vi "SVN_Info_SingleLogEntry_ParseCMDOutput.vi"(8 "Error In":errorcluster, 11 "SVN_Log_XML (In)":string="<?xml version=\"1.0\" encoding=\"UTF-8\"?>\r\n<log>\r\n<logentry\r\n   revision=\"23\">\r\n<author>Admin</author>\r\n<date>2018-04-07T20:16:29.107705Z</date>\r\n<msg></msg>\r\n</logentry>\r\n<logentry\r\n   revision=\"22\">\r\n<author>Admin</author>\r\n<date>2018-04-07T20:12:54.923454Z</date>\r\n<msg></msg>\r\n</logentry>\r\n<logentry\r\n   revision=\"21\">\r\n<author>Admin</author>\r\n<date>2018-04-07T20:12:03.070489Z</date>\r\n<msg></msg>\r\n</logentry>\r\n<logentry\r\n   revision=\"20\">\r\n<author>Marvin</author>\r\n<date>2017-12-05T21:00:12.256074Z</date>\r\n<msg></msg>\r\n</logentry>\r\n<logentry\r\n   revision=\"17\">\r\n<author>Marvin</author>\r\n<date>2017-12-05T20:36:10.326601Z</date>\r\n<msg>10k LoadSpeedTest\r\n</msg>\r\n</logentry>\r\n<logentry\r\n   revision=\"16\">\r\n<author>Marvin</author>\r\n<date>2017-07-06T14:47:03.129259Z</date>\r\n<msg></msg>\r\n</logentry>\r\n<logentry\r\n   revision=\"11\">\r\n<author>Marvin</author>\r\n<date>2017-07-04T16:12:46.837966Z</date>\r\n<msg></msg>\r\n</logentry>\r\n<logentry\r\n   revision=\"7\">\r\n<author>Marvin</author>\r\n<date>2017-07-04T16:05:39.382517Z</date>\r\n<msg></msg>\r\n</logentry>\r\n<logentry\r\n   revision=\"6\">\r\n<author>Marvin</author>\r\n<date>2017-07-04T16:05:05.356571Z</date>\r\n<msg></msg>\r\n</logentry>\r\n<logentry\r\n   revision=\"3\">\r\n<author>Marvin</author>\r\n<date>2017-07-04T15:57:28.132419Z</date>\r\n<msg></msg>\r\n</logentry>\r\n<logentry\r\n   revision=\"1\">\r\n<author>Marvin</author>\r\n<date>2017-07-04T15:51:57.071483Z</date>\r\n<msg>Imported folder structure</msg>\r\n</logentry>\r\n</log>\r\n") -> (0 "Error Out":errorcluster, 3 "SVN_Info_Cluster":T1)   [LabVIEW 2014]
uses:
  <resource>/objmgr/DOMUserDefRef.rc
  <vilib>/xml/NI_XML.lvlib
  <vilib>/xml/Load XML String.vi
  controls/SVN_LogEntry_Cluster.ctl
  controls/SVN_Info_Cluster.ctl
  <vilib>/xml/Close Reference(Node).vi
panel:
  out "commit node values this.Ver":string[](array[string])
  out "commit values this.Ver":string[](array[string])
  out "Attributes":string
  in  "XML String":string="<node_1>\n <node_2 name = \"second_node\"> text </node_2>\n <node_3 type = \"a\"> \n<node_4> text </node_4>\n </node_3>\n</node_1>"
  out "entry values HEAD":string[](array[string])
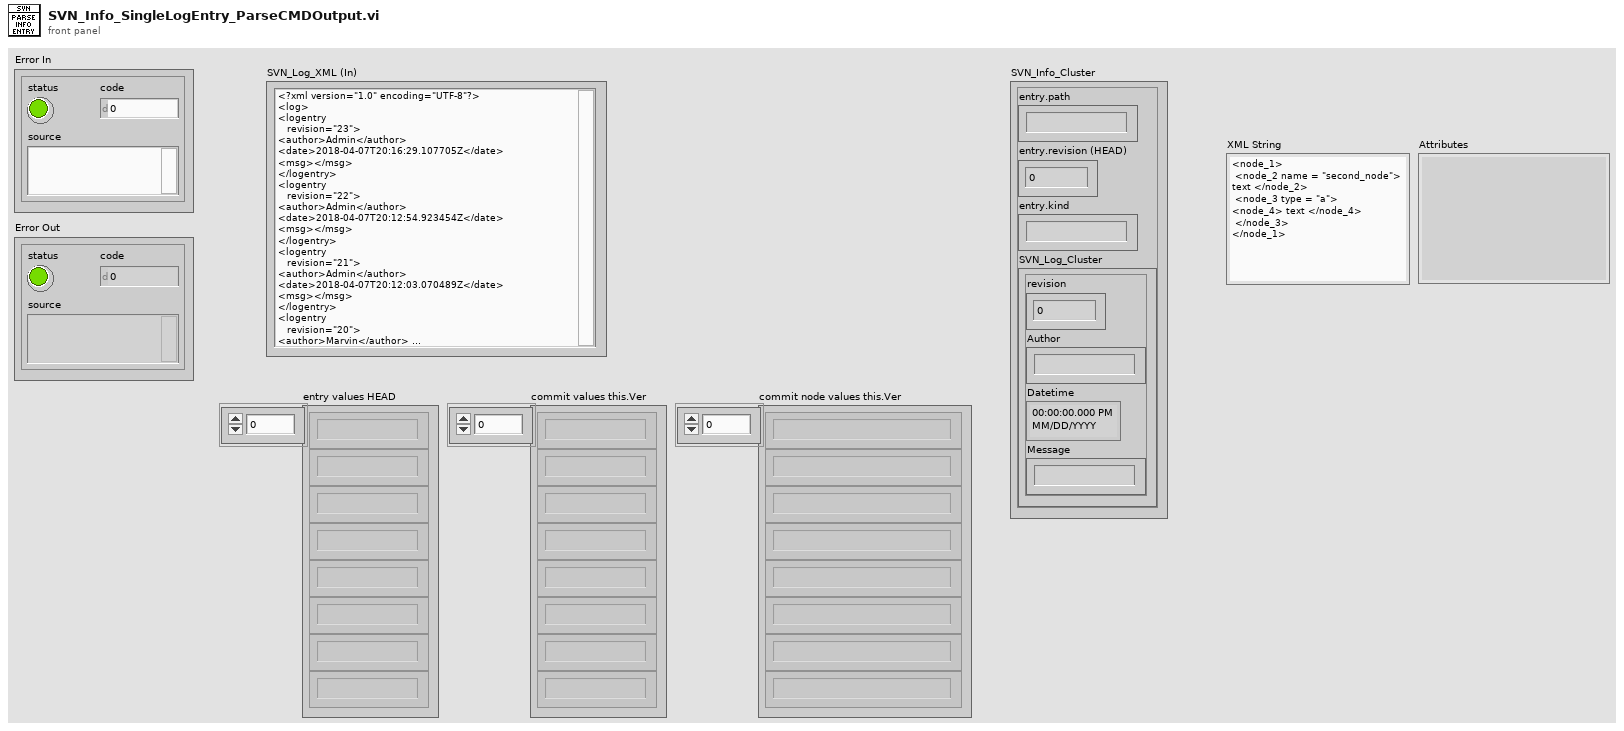
[diagram p1: front panel]
types:
  T1 = typedef "SVN_Info_Cluster.ctl" = cluster{"entry.path":string, "entry.revision (HEAD)":i32, "entry.kind":string, "SVN_Log_Cluster":T2}
  T2 = typedef "SVN_LogEntry_Cluster.ctl" = cluster{"revision":i32, "Author":string, "Datetime":timestamp, "Message":string}
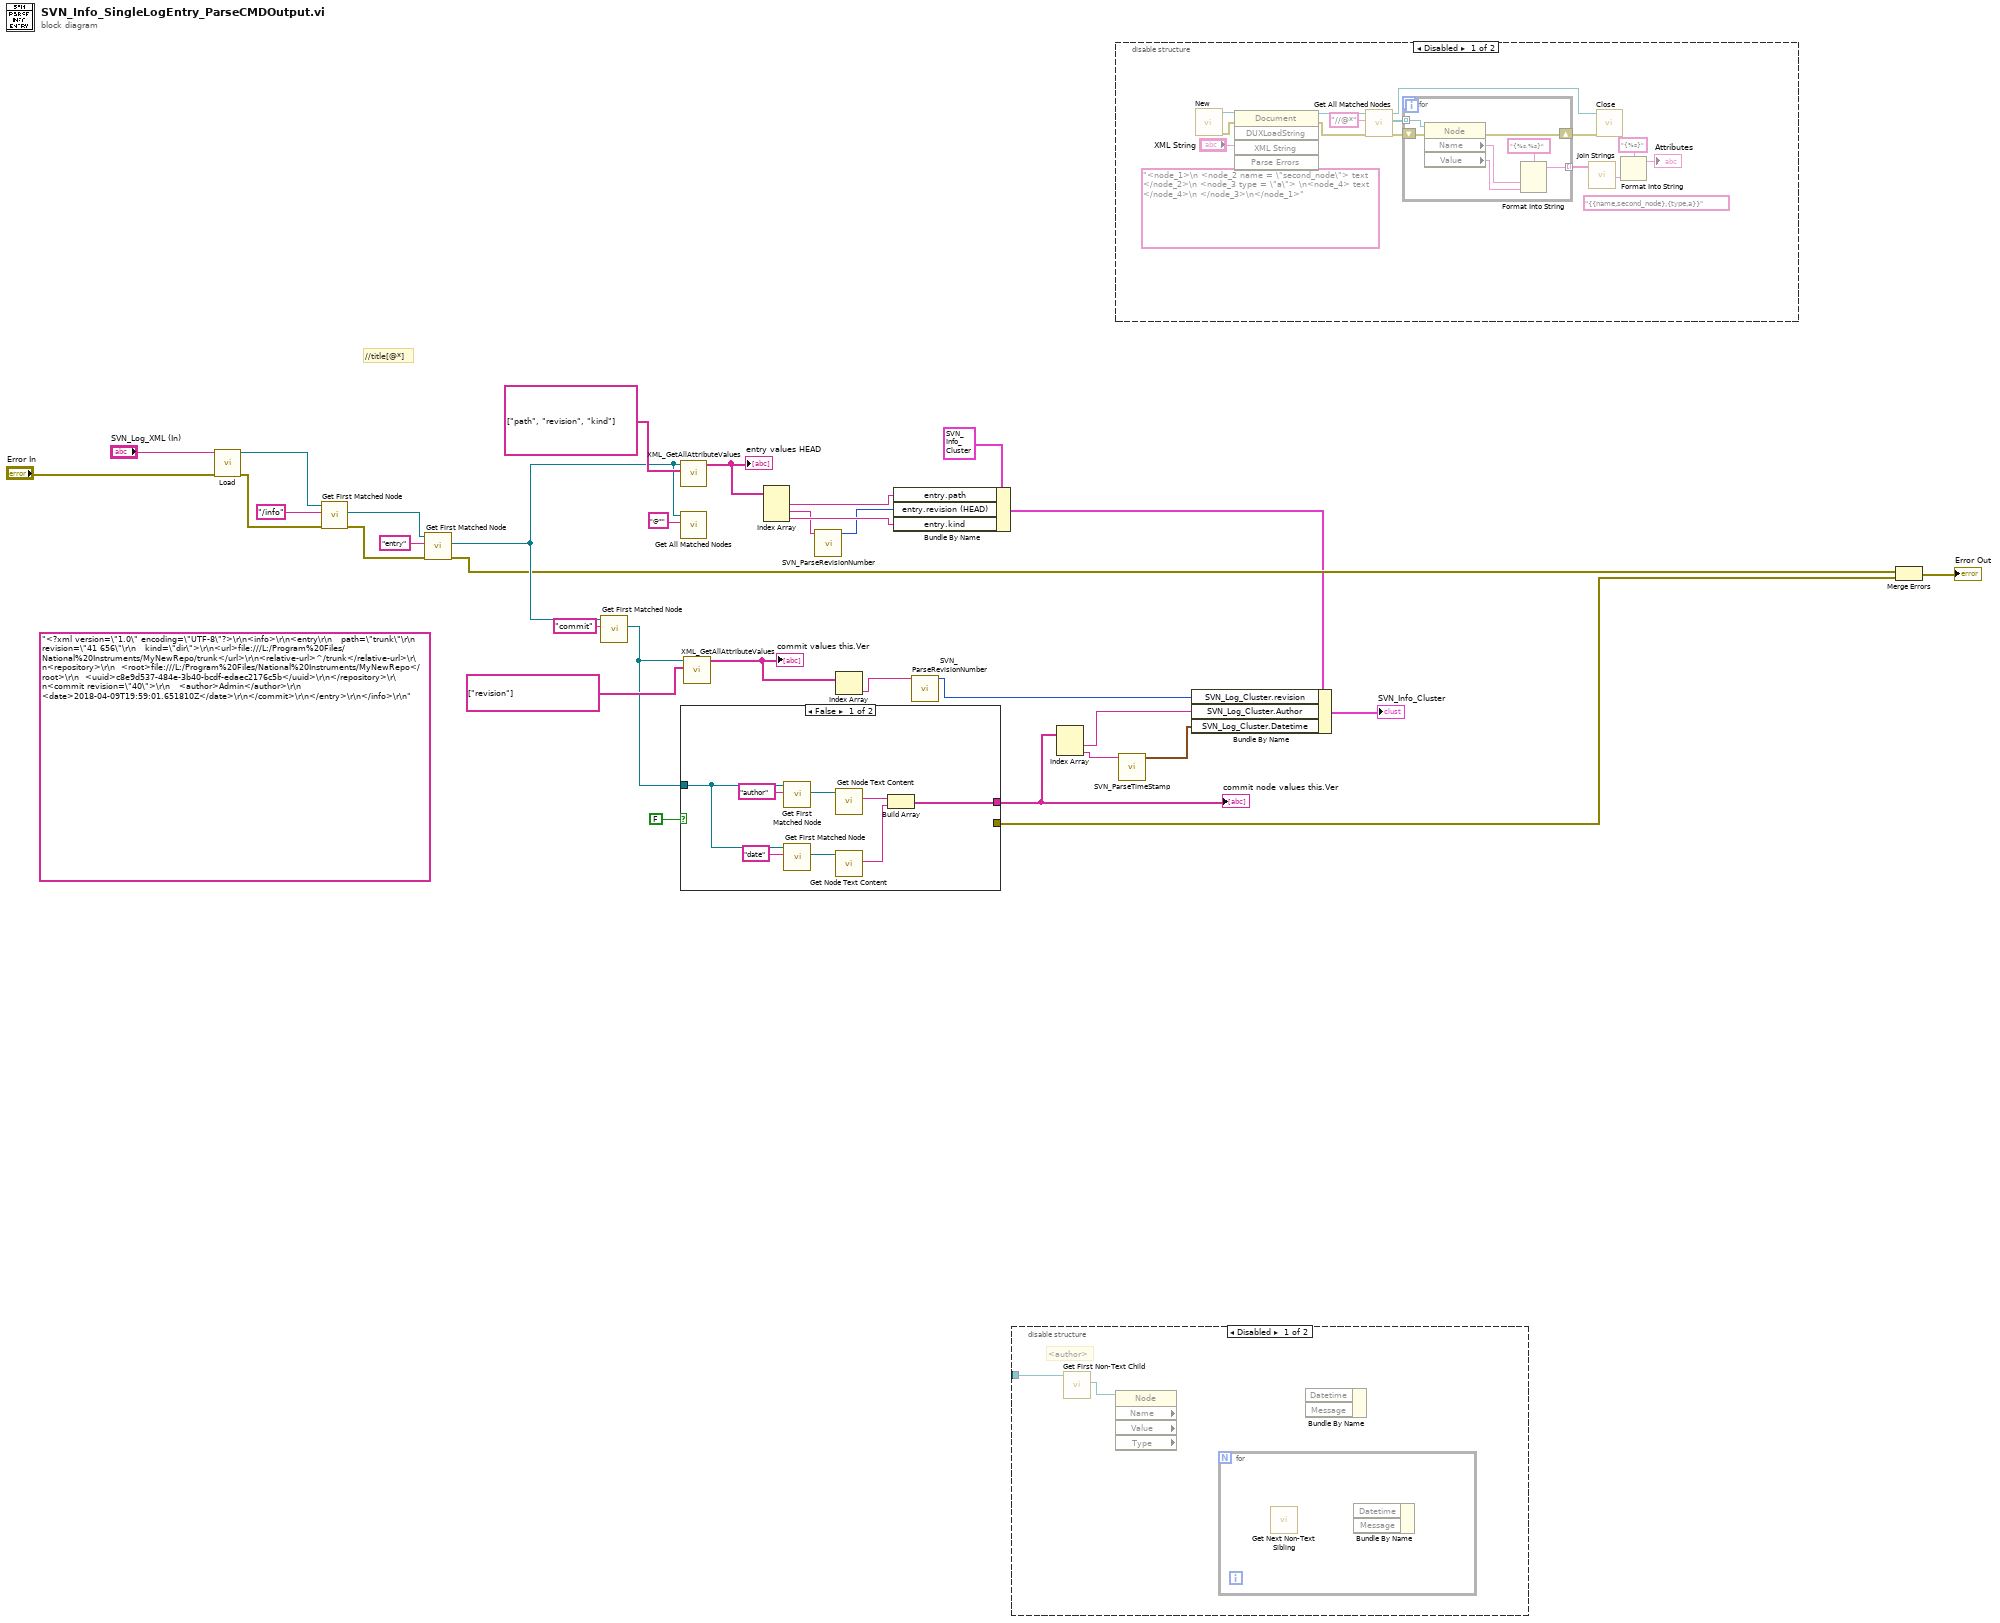
[diagram p0: block diagram]
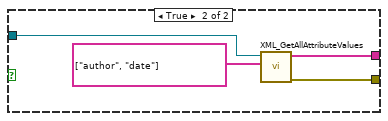
[diagram p2: hidden frame]
diagram:
  (unwired) "<?xml version=\"1.0\" encoding=\"UTF-8\"?>\r\n<info>\r\n<entry\r\n   path=\"trunk\"\r\n   revision=\"41 656\"\r\n   kind=\"dir\">\r\n<url>file:///L:/Program%20Files/National%20Instruments/MyNewRepo/trunk</url>\r\n<relative-url>^/trunk</relative-url>\r\n<repository>\r\n  <root>file:///L:/Program%20Files/National%20Instruments/MyNewRepo</root>\r\n  <uuid>c8e9d537-484e-3b40-bcdf-edaec2176c5b</uuid>\r\n</repository>\r\n<commit revision=\"40\">\r\n   <author>Admin</author>\r\n   <date>2018-04-09T19:59:01.651810Z</date>\r\n</commit>\r\n</entry>\r\n</info>\r\n"
  # "//title[@*]"
  n1 = call-poly <vilib>:"Load.vi"("XML string"="SVN_Log_XML (In)", "error in (no error)"="Error In") -> ("DOM document out"=w27:refnum<k20>, "error out"=w30:errorcluster)  [unwired: 11 in, 1 out]
  n2 = call <vilib>:"Get First Matched Node.vi"("error in (no error)"=w30, "XPath expression"="/info", "node in"=w27) -> ("error out"=w17:errorcluster, "node result"=w23:refnum<k20>)  [unwired: 6 in, 1 out]
  n3 = call <vilib>:"Get First Matched Node.vi"("error in (no error)"=w17, "XPath expression"="entry", "node in"=w23) -> ("error out"=w18:errorcluster, "node result"=w19:refnum<k20>)  [unwired: 6 in, 1 out]
  n4 = call <vilib>:"Get First Matched Node.vi"("XPath expression"="commit", "node in"=w19) -> ("node result"=w21:refnum<k20>)  [unwired: 7 in, 2 out]
  n5 = call "XML_GetAllAttributeValues.vi"("Attribute Names to find[]"=string[] ["path", "revision", "kind"], "Node Refnum (In)"=w19) -> ("Attribute Values[]"=w11:string[])  [unwired: 8 in, 1 out]
  "entry values HEAD" <- w11
  n6 = call <vilib>:"Get All Matched Nodes.vi"("XPath expression"="@*", "node in"=w19) -> ()  [unwired: 7 in, 3 out]
  n7 = case shown="False" FALSE {
    tunnel: w21 -> [w39 w45]
    tunnel: [w34 w44] -> w15
    tunnel: [_ w42] -> w20
    frame False {
      n8 = call <vilib>:"Get First Matched Node.vi"("XPath expression"="author", "node in"=w39) -> ("node result"=w38:refnum<k20>)  [unwired: 7 in, 2 out]
      n9 = call <vilib>:"Get First Matched Node.vi"("XPath expression"="date", "node in"=w39) -> ("node result"=w37:refnum<k20>)  [unwired: 7 in, 2 out]
      n10 = call <vilib>:"Get Node Text Content.vi"("node in"=w38) -> ("node text"=w36:string)  [unwired: 8 in, 2 out]
      n11 = call <vilib>:"Get Node Text Content.vi"("node in"=w37) -> ("node text"=w35:string)  [unwired: 8 in, 2 out]
      n12 = Build Array(w36, w35) -> (w34:string[])
    }
    frame True {
      n13 = call "XML_GetAllAttributeValues.vi"("Attribute Names to find[]"=string[] ["author", "date"], "Node Refnum (In)"=w45) -> ("Error Out"=w42:errorcluster, "Attribute Values[]"=w44:string[])  [unwired: 8 in]
    }
  }
  "commit node values this.Ver" <- w15
  n14 = call "XML_GetAllAttributeValues.vi"("Attribute Names to find[]"=string[] ["revision"], "Node Refnum (In)"=w21) -> ("Attribute Values[]"=w5:string[])  [unwired: 8 in, 1 out]
  "commit values this.Ver" <- w5
  n15 = Index Array(array=w11) -> (element #1=w9:string, element #2=w8:string, element #3=w10:string)  [unwired: 3 in]
  n16 = call "SVN_ParseRevisionNumber.vi"("rev str (In)"=w8) -> ("number"=w7:i32)  [unwired: 10 in]
  n17 = Index Array(array=w5) -> (element=w4:string)  [unwired: 1 in]
  n18 = Bundle By Name(cluster=T1 {"entry.path"="", "entry.revision (HEAD)"=0, "entry.kind"="", "SVN_Log_Cluster"={"revision"=0, "Author"="", "Datetime"=timestamp(0 s since 1904-01-01), "Message"=""}} ("SVN_Info_Cluster"), "entry.path"=w9, "entry.revision (HEAD)"=w7, "entry.kind"=w10) -> (w13:T1)
  n19 = call "SVN_ParseRevisionNumber.vi"("rev str (In)"=w4) -> ("number"=w3:i32)  [unwired: 10 in]
  n20 = disable-structure shown="Disabled" {
    disable-tunnel: _ -> [w47 _]
    frame Disabled {
      # "<author>"
      n21 = call <vilib>:"Get First Non-Text Child.vi"("node in"=w47) -> ("child node"=w46:refnum<k20>)  [unwired: 7 in, 3 out]
      n22 = property class="Node" props=["Name", "Value", "Type"](reference=w46) -> ()  [unwired: 1 in, 5 out]
      n23 = for {
        n24 = call <vilib>:"Get Next Non-Text Sibling.vi"() -> ()  [unwired: 8 in, 4 out]
        n25 = Bundle By Name() -> ()  [unwired: 3 in, 1 out]
      }
      n26 = Bundle By Name() -> ()  [unwired: 3 in, 1 out]
    }
    frame Enabled {
    }
  }
  n27 = Index Array(array=w15) -> (element #1=w2:string, element #2=w14:string)  [unwired: 2 in]
  n28 = disable-structure shown="Disabled" {
    frame Disabled {
      (unwired) "<node_1>\n <node_2 name = \"second_node\"> text </node_2>\n <node_3 type = \"a\"> \n<node_4> text </node_4>\n </node_3>\n</node_1>" ("XML String")
      (unwired) "{{name,second_node},{type,a}}" ("Attributes")
      n29 = call <vilib>:"New.vi"() -> ("error out"=w59:errorcluster, "DOM document out"=w60:refnum<k20>)  [unwired: 8 in]
      n30 = invoke class="Document" method="DUXLoadString"(reference=w60, error in=w59, "XML String"="XML String") -> (reference out=w58:refnum<k20>, error out=w57:errorcluster)  [unwired: 2 in, 3 out]
      n31 = call <vilib>:"Get All Matched Nodes.vi"("error in (no error)"=w57, "XPath expression"="//@*", "node in"=w58) -> ("error out"=w54:errorcluster, "node result array"=w55:refnum<k20>[], "node out"=w48:refnum<k20>)  [unwired: 6 in]
      n32 = for {
        tunnel: w55 -> [w66] mode=indexing
        shift-right: [w67] -> w49
        shift-left: w54 -> [w68]
        tunnel: [w62] -> w53 mode=indexing
        n33 = property class="Node"(reference=w66, error in=w68) -> (error out=w67:errorcluster, "Name"=w65:string, "Value"=w64:string)  [unwired: 1 out]
        n34 = Format Into String(format string="{%s,%s}", w65, w64) -> (resulting string=w62:string)  [unwired: 2 in, 1 out]
      }
      n35 = call <vilib>:"Join Strings.vi"("Strings In"=w53) -> ("String"=w52:string)  [unwired: 2 in]
      n36 = call-poly <vilib>:"Close.vi"("error in (no error)"=w49, "node"=w48) -> ()  [unwired: 7 in, 1 out]
      n37 = Format Into String(format string="{%s}", w52) -> (resulting string=→"Attributes":string)  [unwired: 2 in, 1 out]
    }
    frame Enabled {
    }
  }
  n38 = call "SVN_ParseTimeStamp.vi"("Timestring (In)"=w14) -> ("Timestamp (Out)"=w6:timestamp)  [unwired: 10 in]
  n39 = Bundle By Name(cluster=w13, "SVN_Log_Cluster.revision"=w3, "SVN_Log_Cluster.Author"=w2, "SVN_Log_Cluster.Datetime"=w6) -> (→"SVN_Info_Cluster":T1)
  n40 = Merge Errors(w18, w20) -> (→"Error Out":errorcluster)
